vi "ConfigUtilities - Clear Listbox Delete Indices.vi"(7 "Listbox Reference in":refnum<vi>, 8 "error in (no error)":errorcluster, 9 "Pane Coords":T1, 10 "Delete Property Name":string, 11 "Item Ref in":T2 format="%.0x") -> (0 "error out":errorcluster, 3 "Listbox Reference out":refnum<vi>)   [LabVIEW 2016, in "UDP-Custom-Device System Explorer.lvlib"]
uses:
  UDP-Custom-Device System Explorer.lvlib
  <vilib>/NI Veristand/Custom Device API/Custom Device Item Ref.ctl
  <vilib>/Utility/miscctls.llb/LVPoint32TypeDef.ctl
  <vilib>/NI Veristand/Custom Device API/Set Item Property (I32 Array).vi
  <vilib>/NI VeriStand/Custom Device API/Custom Device API.lvlib
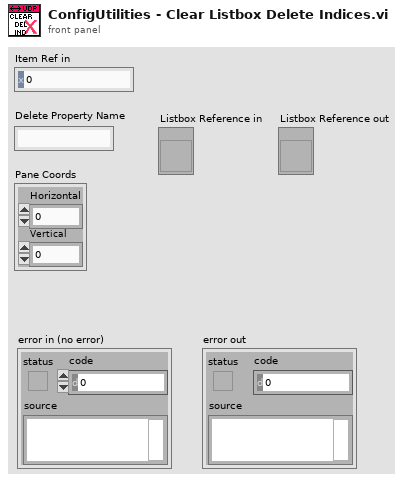
[diagram p1: front panel]
types:
  T1 = typedef "LVPoint32TypeDef.ctl" = cluster{"Horizontal":i32, "Vertical":i32}
  T2 = typedef "Custom Device API.lvlib/Custom Device Item Ref.ctl" = u64
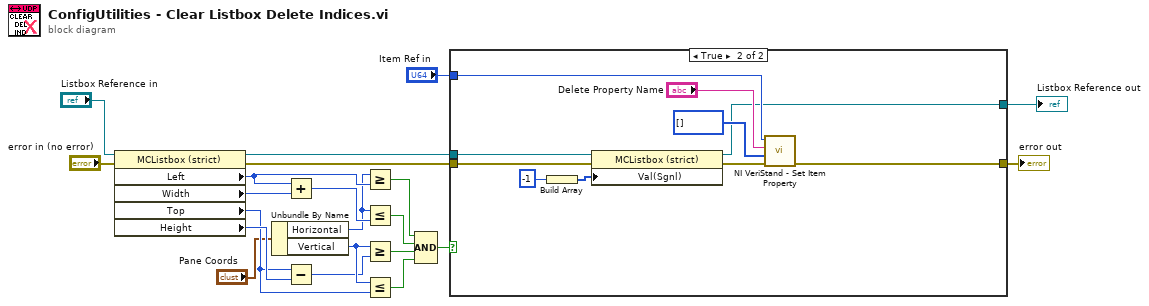
[diagram p0: block diagram]
diagram:
  n1 = property class="MCListbox (strict)"(reference="Listbox Reference in", error in="error in (no error)") -> (reference out=w21:refnum<vi>, error out=w20:errorcluster, "Left"=w15:i32, "Width"=w16:u32, "Top"=w17:i32, "Height"=w18:u32)
  n2 = Unbundle By Name("Pane Coords") -> ("Horizontal"=w4:i32, "Vertical"=w7:i32)
  n3 = Add(x=w15, y=w16) -> (x+y=w5:u32)
  n4 = Subtract(x=w17, y=w18) -> (x-y=w6:u32)
  n5 = Greater Or Equal?(x=w4, y=w15) -> (x >= y?=w8:bool)
  n6 = Less Or Equal?(x=w4, y=w5) -> (x <= y?=w9:bool)
  n7 = Greater Or Equal?(x=w7, y=w6) -> (x >= y?=w10:bool)
  n8 = Less Or Equal?(x=w7, y=w17) -> (x <= y?=w11:bool)
  n9 = Compound Arithmetic op=AND(w8, w9, w10, w11) -> (w12:bool)
  n10 = case shown="True" w12 {
    tunnel: w20 -> [w23 w26]
    tunnel: [w23 w24] -> w13
    tunnel: "Item Ref in" -> [_ w32]
    tunnel: w21 -> [w22 w30]
    tunnel: [w22 w27] -> w1
    frame False {
    }
    frame True {
      n11 = Build Array(-1) -> (w29:i32[])
      n12 = property class="MCListbox (strict)"(reference=w30, error in=w26, "Val(Sgnl)"=w29) -> (reference out=w27:refnum<vi>, error out=w25:errorcluster)
      n13 = call-poly <vilib>:"NI VeriStand - Set Item Property.vi"("error in (no error)"=w25, "Value"=i32[] [], "Property Name"="Delete Property Name", "Item Ref in"=w32) -> ("error out"=w24:errorcluster)  [unwired: 5 in, 2 out]
    }
  }
  "error out" <- w13
  "Listbox Reference out" <- w1
